vi "MH_InitDone.vi"(8 "error in (no error)":errorcluster, 9 "MH Init Info":cluster{"DevIdx":i32, "Init Info":T1}, 10 "InstrumentData":T2, 11 "MultiharpComm in":refnum<class "MultiharpComm.lvclass">) -> (0 "error out":errorcluster, 3 "MultiharpComm out":refnum<class "MultiharpComm.lvclass">)   [LabVIEW 2023, in "MultiharpComm.lvlib" / "MultiharpComm.lvclass"]
uses:
  MultiharpComm.lvclass
  typedefs/instrumentType.ctl
  typedefs/typedefs.lvlib
  typedefs/InstrumentData.ctl
  Multiharp/_lib/PQ/MultiHarp/MH_InitInfo.ctl
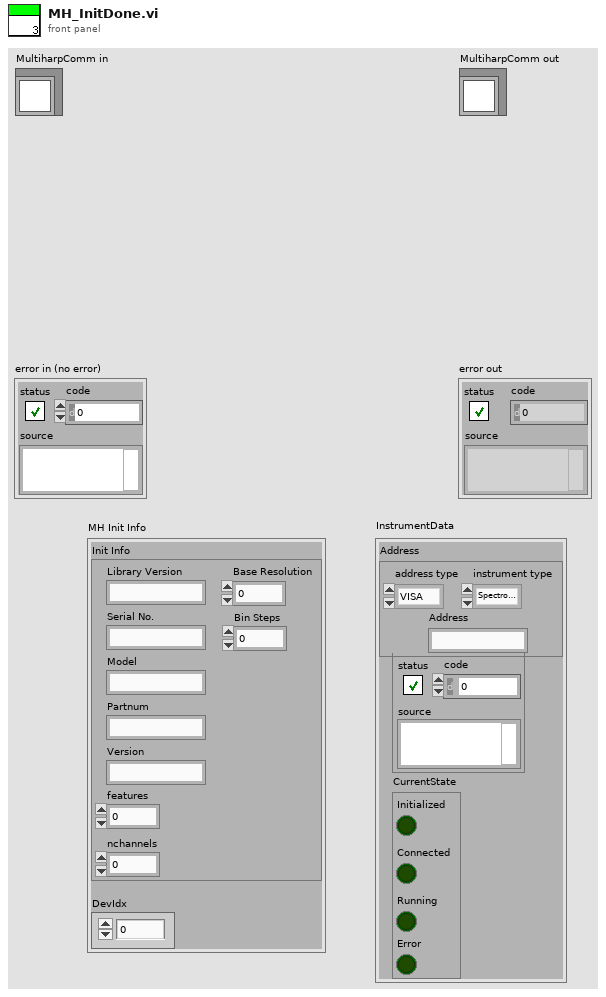
[diagram p1: front panel]
types:
  T1 = typedef "typedefs.lvlib/MH_InitInfo.ctl" = cluster{"Library Version":string, "Serial No.":string, "Model":string, "Partnum":string, "Version":string, "features":i32, "nchannels":i32, "Base Resolution":dbl, "Bin Steps":i32}
  T2 = typedef "typedefs.lvlib/InstrumentData.ctl" = cluster{"Instr Error":errorcluster, "Address":cluster{"address type":enum16{"VISA", "Index"}, "Address":string, "instrument type":T3}, "CurrentState":cluster{"Initialized":bool, "Connected":bool, "Running":bool, "Error":bool}}
  T3 = typedef "typedefs.lvlib/instrumentType.ctl" = enum16{"Spectrometer", "Camera", "Stepper", "Piezo", "SLM"}
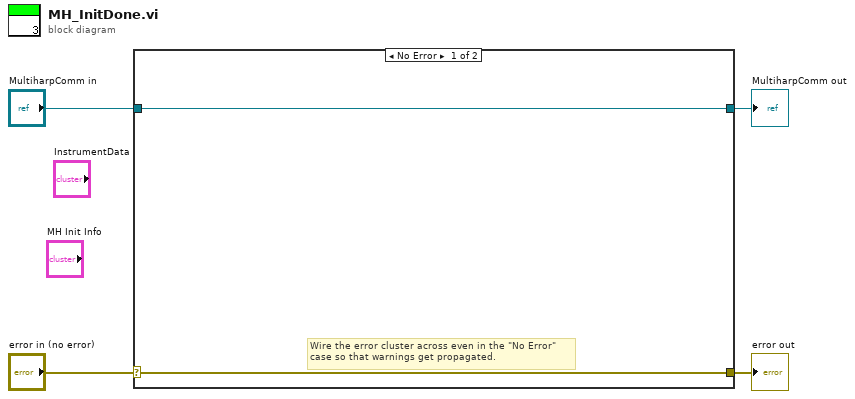
[diagram p0: block diagram]
diagram:
  n1 = case shown="No Error" "error in (no error)" {
    selector: "error in (no error)" -> [w5 w8]
    tunnel: [w5 w8] -> w3
    tunnel: [w6 w7] -> w1
    tunnel: "MultiharpComm in" -> [w6 w7]
    frame No Error {
      # "Wire the error cluster across even in the \"No Error\"\ncase so that warnings get propagated."
    }
    frame Error {
    }
  }
  "error out" <- w3
  "MultiharpComm out" <- w1
